vi "KeeperDefPosSkillVSS.vi"(8 "error in (no error)":errorcluster, 9 "Game":refnum<class "Game.lvclass">, 10 "Robot in":refnum<class "Robot.lvclass">, 11 "KeeperDefPosSkillVSS in":refnum<class "KeeperDefPosSkillVSS.lvclass">) -> (0 "error out":errorcluster, 2 "Robot out":refnum<class "Robot.lvclass">, 3 "KeeperDefPosSkillVSS out":refnum<class "KeeperDefPosSkillVSS.lvclass">)   [LabVIEW 2020, in "KeeperDefPosSkillVSS.lvclass"]
uses:
  KeeperDefPosSkillVSS.lvclass
  Robot_class/Robot.lvclass
  C:/ROBOIME/SSL_AI/Object_class/Object.lvclass
  Game_class/Game.lvclass
  Game_class/Game.lvclass/Game.ctl
  Ball_class/Ball.lvclass/Ball.ctl
  Object_class/Object.lvclass/Object.ctl
  Robot_class/Robot.lvclass/Robot.ctl
  Object_class/Read y.vi
  Game_class/Read FieldRef.vi
  Game_class/Read BallRef.vi
  Ball_class/Read v_x.vi
  Ball_class/Read v_y.vi
  Object_class/Read x.vi
  Robot_class/Write dest_x.vi
  Robot_class/Write dest_y.vi
  Robot_class/Write dest_orientation.vi
  Ball_class/Ball.lvclass
  Field_class/Field.lvclass
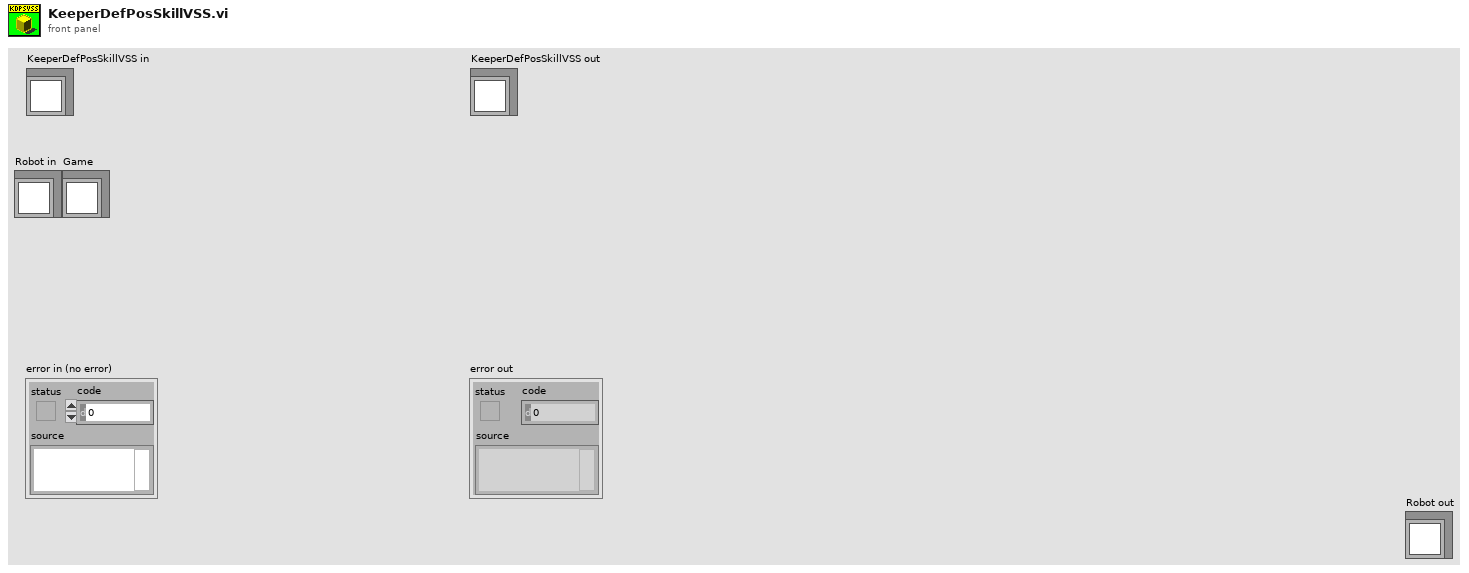
[diagram p1: front panel]
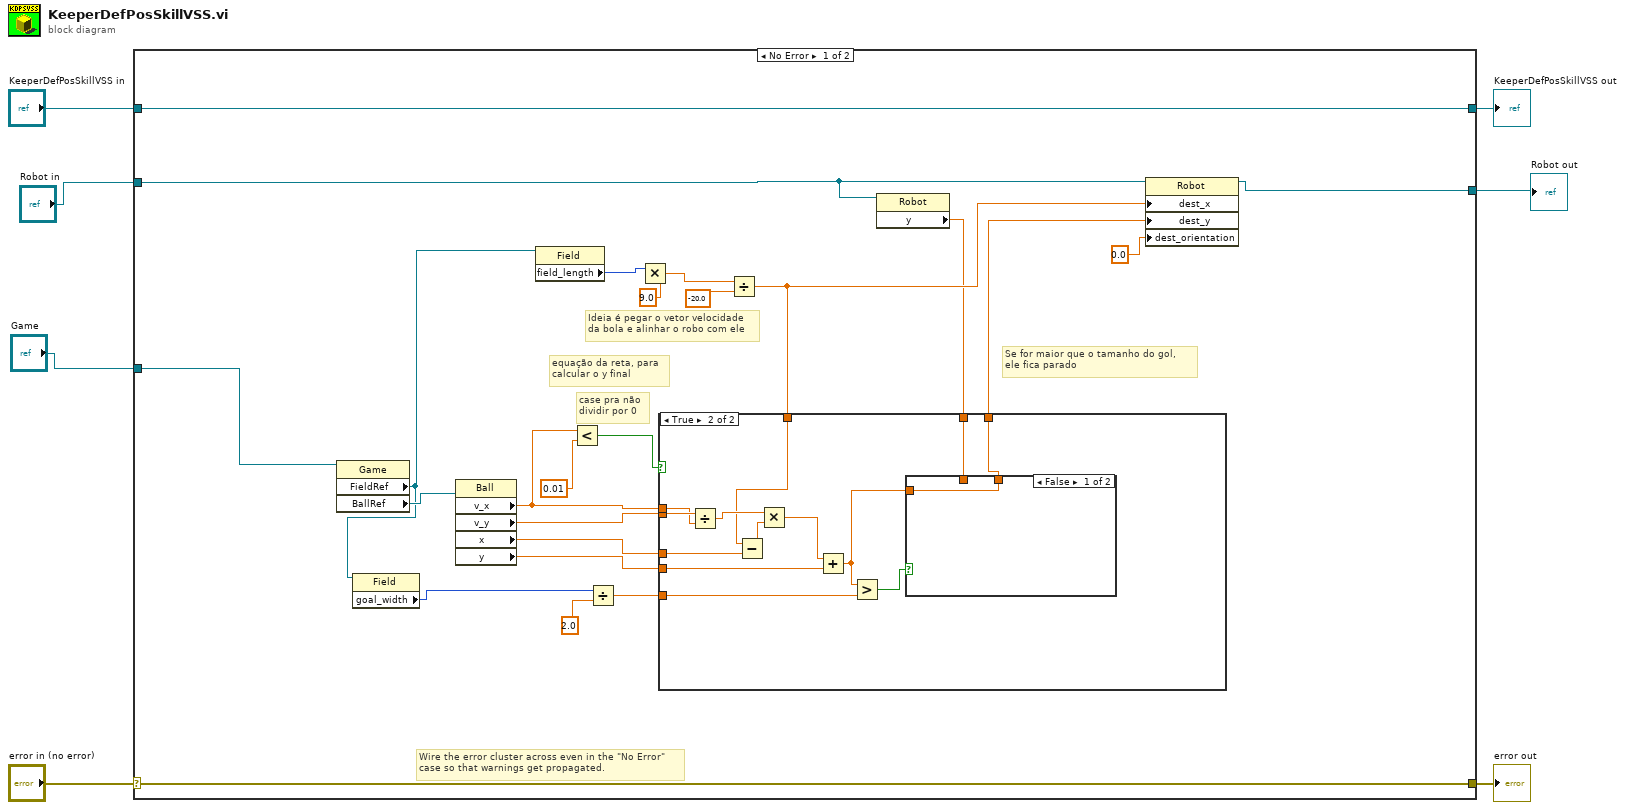
[diagram p0: block diagram]
diagram:
  n1 = case shown="No Error" "error in (no error)" {
    selector: "error in (no error)" -> [w30 w50]
    tunnel: [w30 w50] -> w6
    tunnel: [w31 w49] -> w4
    tunnel: "KeeperDefPosSkillVSS in" -> [w31 w49]
    tunnel: "Game" -> [w13 _]
    tunnel: "Robot in" -> [w12 w48]
    tunnel: [w11 w48] -> w1
    frame No Error {
      # "case pra não \ndividir por 0"
      # "Se for maior que o tamanho do gol, \nele fica parado"
      # "equação da reta, para \ncalcular o y final"
      # "Ideia é pegar o vetor velocidade \nda bola e alinhar o robo com ele"
      # "Wire the error cluster across even in the \"No Error\"\ncase so that warnings get propagated."
      n2 = property class="Game"(reference=w13) -> ("FieldRef"=w19:refnum<class "Field.lvclass">, "BallRef"=w29:refnum<class "Ball.lvclass">)  [unwired: 1 in, 2 out]
      n3 = property class="Field"(reference=w19) -> ("goal_width"=w18:i32)  [unwired: 1 in, 2 out]
      n4 = property class="Ball"(reference=w29) -> ("v_x"=w10:dbl, "v_y"=w23:dbl, "x"=w22:dbl, "y"=w20:dbl)  [unwired: 1 in, 2 out]
      n5 = property class="Field"(reference=w19) -> ("field_length"=w28:i32)  [unwired: 1 in, 2 out]
      n6 = Less?(x=w10, y=0.01) -> (x < y?=w8:bool)
      n7 = Divide(x=w18, y=2.0) -> (x/y=w16:dbl)
      n8 = Multiply(x=w28, y=9.0) -> (x*y=w25:dbl)
      n9 = Divide(x=w25, y=-20.0) -> (x/y=w21:dbl)
      n10 = property class="Robot"(reference=w12) -> ("y"=w14:dbl)  [unwired: 1 in, 2 out]
      n11 = case shown="True" w8 {
        tunnel: w23 -> [_ w45]
        tunnel: w22 -> [_ w43]
        tunnel: w21 -> [_ w42]
        tunnel: w20 -> [_ w40]
        tunnel: w16 -> [_ w38]
        tunnel: [w32 w36] -> w15
        tunnel: w14 -> [w32 w35]
        tunnel: w10 -> [_ w33]
        frame False {
        }
        frame True {
          n12 = Divide(x=w45, y=w33) -> (x/y=w44:dbl)
          n13 = Subtract(x=w42, y=w43) -> (x-y=w41:dbl)
          n14 = Multiply(x=w44, y=w41) -> (x*y=w39:dbl)
          n15 = Add(x=w39, y=w40) -> (x+y=w34:dbl)
          n16 = Greater?(x=w34, y=w38) -> (0:w37:bool)
          n17 = case shown="False" w37 {
            tunnel: [w46 w47] -> w36
            tunnel: w35 -> [_ w47]
            tunnel: w34 -> [w46 _]
            frame False {
            }
            frame True {
            }
          }
        }
      }
      n18 = property class="Robot"(reference=w12, "dest_x"=w21, "dest_y"=w15, "dest_orientation"=0.0) -> (reference out=w11:refnum<class "Robot.lvclass">)  [unwired: 1 in, 1 out]
    }
    frame Error {
    }
  }
  "error out" <- w6
  "KeeperDefPosSkillVSS out" <- w4
  "Robot out" <- w1
